vi "rx metadata strerror.vi"(8 "error in (no error)":errorcluster, 9 "strbuffer_len":u64, 10 "strerror_out":string, 11 "h":u64) -> (0 "error out":errorcluster, 1 "function return":u32(ring), 2 "strerror_out out":string, 3 "h out":u64)   [LabVIEW 2023, in "uhd.lvlib"]
doc: "UHD_API uhd_error uhd_rx_metadata_strerror(\n uhd_rx_metadata_handle h, char* strerror_out, size_t strbuffer_len);"
uses:
  <userlib>/uhd/uhd.lvlib
  <userlib>/uhd/uhd.dll
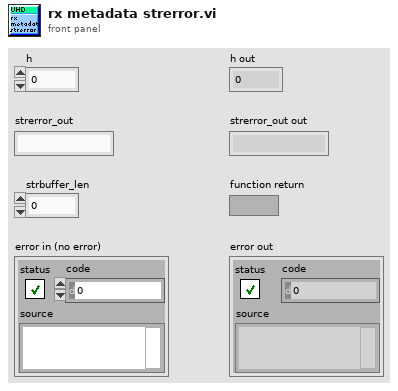
[diagram p1: front panel]
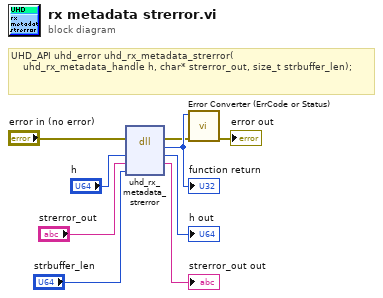
[diagram p0: block diagram]
diagram:
  # "UHD_API uhd_error uhd_rx_metadata_strerror(\n    uhd_rx_metadata_handle h, char* strerror_out, size_t strbuffer_len);"
  n1 = dll-call lib="C:/Program Files/National Instruments/LabVIEW 2023/user.lib/uhd/uhd.*" fn="uhd_rx_metadata_strerror"(error in="error in (no error)", "h"="h", "strerror_out"="strerror_out", "strbuffer_len"="strbuffer_len") -> (error out=w2:errorcluster, w9:u32, "h"=→"h out":u64, "strerror_out"=→"strerror_out out":string)  [unwired: 3 in, 1 out]
  "function return" <- w9
  n2 = call <userlib>:"Error Converter (ErrCode or Status).vi"("error in (no error)"=w2, "error code"=w9) -> ("error out"=→"error out":errorcluster)  [unwired: 9 in]
